vi "UMLEditor_TargetDialog.vi"(6 "SetLastSearchPath(True)":bool=TRUE, 8 "error in (no error)":errorcluster, 10 "Target":string, 11 "GetProjectRefByName":string) -> (0 "error out":errorcluster, 1 "ProjectFolder":path=path "C:/GDS_Test/2009_RT/Test", 2 "ProjectPath":path=path "C:/GDS_Test/2009_RT/Test/Test.lvproj", 3 "TargetIndex":u16, 5 "Targets":string[](array[string]))   [LabVIEW 2016]
uses:
  <resource>/Framework/Providers/Open_GDS/UML/UMLEditor/UMLEditor_StoredPathes.ctl
  <resource>/Framework/Providers/Open_GDS/ClassProviders/Common/File/File_StoredPathesActions.ctl
panel:
  in  "Select":bool
  in  "Target":i32(listbox) caption="Target to use"
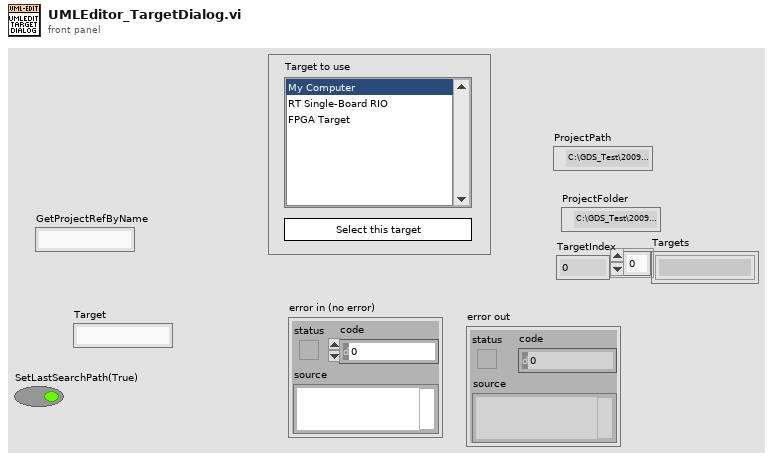
[diagram p1: front panel]
types:
  T1 = typedef "File_StoredPathesActions.ctl" = enum16{"Get Path", "Set Path", "Delete Path", "Clear All Paths"}
  T2 = typedef "UMLEditor_StoredPathes.ctl" = enum16{"LastSearchPath", "QueuedArrayStateVI", "ClassBasePath", "ViTemplatePath", "ApplicationTemplatePath", "IniFilePath", "WizDir", "RevPlugInPath"}
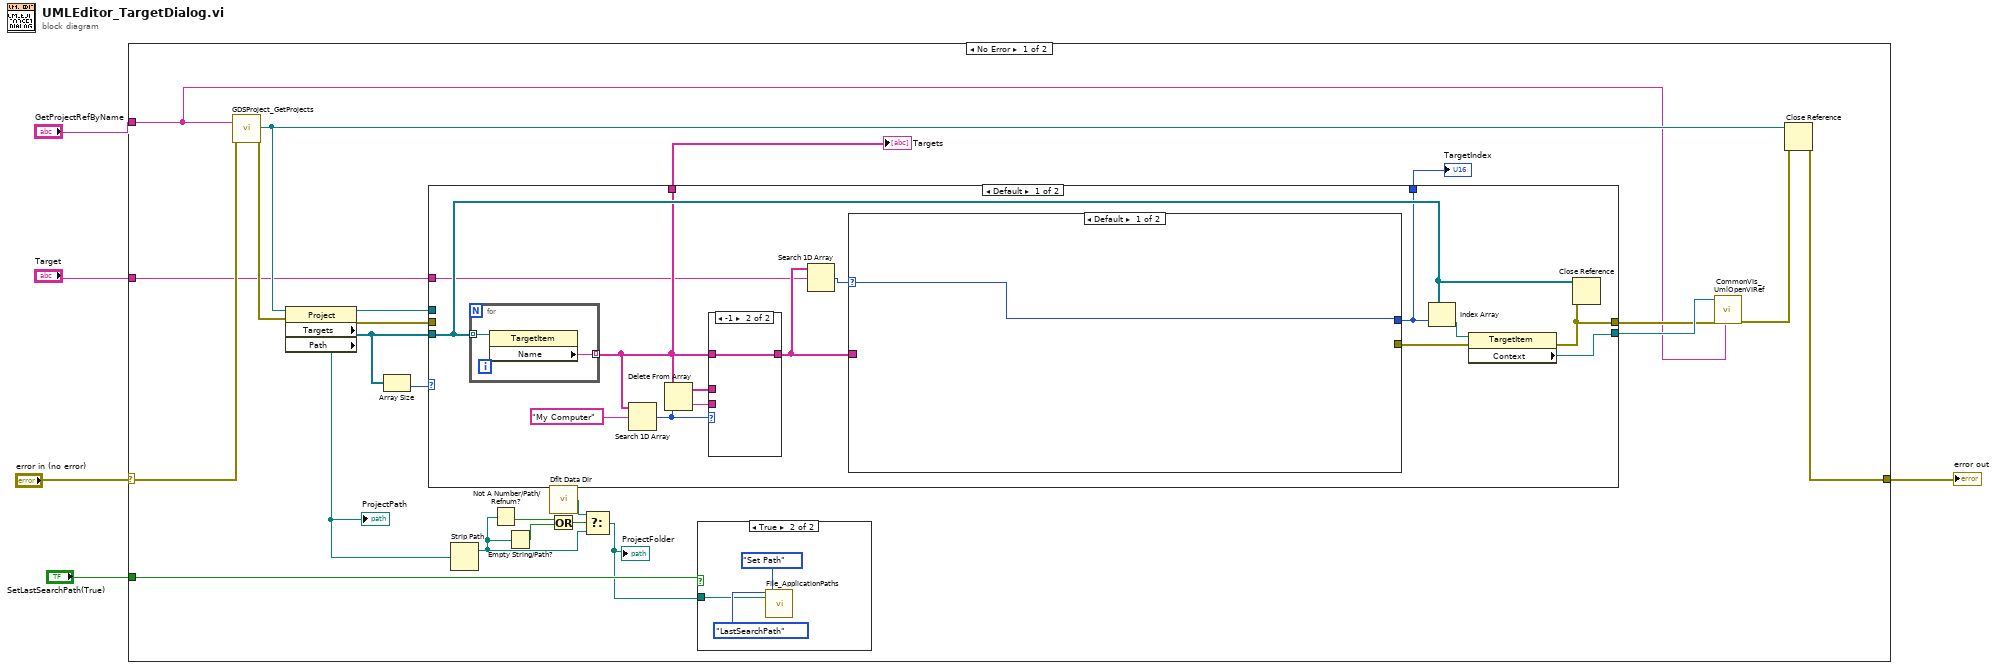
[diagram p0: block diagram]
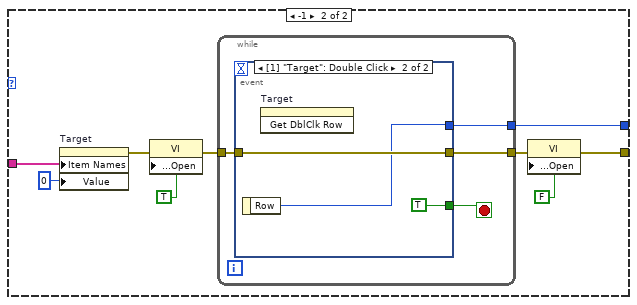
[diagram p3: hidden frame]
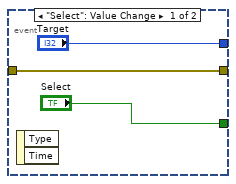
[diagram p4: hidden frame]
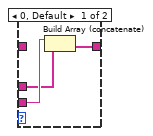
[diagram p5: hidden frame]
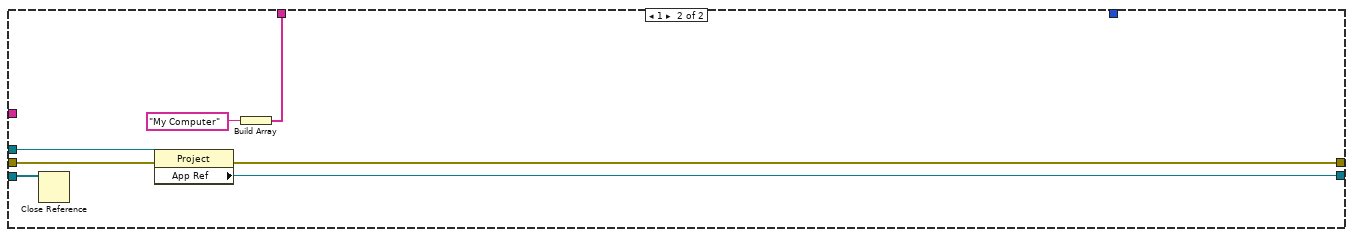
[diagram p6: hidden frame]
diagram:
  n1 = case shown="No Error" "error in (no error)" {
    selector: "error in (no error)" -> [w17 w79]
    tunnel: [w18 w79] -> w5
    tunnel: "GetProjectRefByName" -> [w15 _]
    tunnel: "SetLastSearchPath(True)" -> [w16 _]
    tunnel: "Target" -> [w12 _]
    frame No Error {
      n2 = call <resource>:"GDSProject_GetProjects.vi"("GetProjectRefByName"=w15, "error in (no error)"=w17) -> ("Project Refnum"=w20:refnum<vi>, "error out"=w23:errorcluster)  [unwired: 1 in, 15 out]
      n3 = property class="Project"(reference=w20, error in=w23) -> (reference out=w25:refnum<vi>, error out=w24:errorcluster, "Targets"=w26:refnum<vi>[], "Path"=w19:path)
      "ProjectPath" <- w19
      n4 = Array Size(array=w26) -> (size(s)=w27:i32)
      n5 = case shown="Default" w27 {
        tunnel: w26 -> [w38 w78]
        tunnel: w25 -> [_ w77]
        tunnel: w24 -> [_ w76]
        tunnel: [w40 w75] -> w22
        tunnel: [w39 w74] -> w21
        tunnel: [w36 w72] -> w14
        tunnel: [w35 _] -> w13
        tunnel: w12 -> [w33 _]
        frame Default {
          n6 = for {
            tunnel: w38 -> [w71] mode=indexing
            tunnel: [w70] -> w36 mode=indexing
            n7 = property class="TargetItem"(reference=w71) -> ("Name"=w70:string)  [unwired: 1 in, 2 out]
          }
          n8 = Search 1D Array(1D array=w36, element="My Computer") -> (index of element=w44:i32)  [unwired: 1 in]
          n9 = Delete From Array(array=w36, index=w44) -> (deleted portion=w43:string, array with subset deleted=w37:string[])  [unwired: 1 in]
          n10 = case shown="-1" w44 {
            tunnel: w36 -> [_ w69]
            tunnel: [w67 w69] -> w34
            tunnel: w43 -> [w68 _]
            tunnel: w37 -> [w66 _]
            frame 0, Default {
              n11 = Build Array (concatenate)(w68, w66) -> (w67:string[])
            }
            frame -1 {
            }
          }
          n12 = Search 1D Array(1D array=w34, element=w33) -> (index of element=w32:i32)  [unwired: 1 in]
          n13 = case shown="Default" w32 {
            selector: w32 -> [w46 _]
            tunnel: w34 -> [_ w50]
            tunnel: [_ w48] -> w42
            tunnel: [w46 w47] -> w35
            frame Default {
            }
            frame -1 {
              n14 = property on="Target" class="LstBox (strict)"("Item Names"=w50, "Value"=0 ("Target")) -> (error out=w55:errorcluster)  [unwired: 2 in, 1 out]
              n15 = property class="VI"(error in=w55, "Front Panel.Open"=TRUE ("Front Panel Window:Open")) -> (error out=w53:errorcluster)  [unwired: 1 in, 1 out]
              n16 = while {
                tunnel: w53 -> [w59]
                tunnel: [w58] -> w51
                tunnel: [w57] -> w47
                stop <- w56 stop-if-true
                n17 = event shown="[1] \"Target\": Double Click" {
                  selector: _ -> [_ _]
                  dyn-events: _ -> [_ _]
                  timeout: _ -> [_ _]
                  tunnel: w59 -> [w62 w65]
                  tunnel: [w62 w65] -> w58
                  tunnel: ["Target" w64] -> w57
                  tunnel: ["Select" TRUE ("Select")] -> w56
                  event "Select": Value Change {
                    n18 = event-data() -> ()  [unwired: 1 in, 2 out]
                  }
                  event "Target": Double Click {
                    n19 = event-data() -> ("Row"=w64:i32)  [unwired: 1 in]
                    n20 = invoke on="Target" class="LstBox (strict)" method="Get DblClk Row"() -> ()  [unwired: 3 in, 3 out]
                  }
                }
              }
              n21 = property class="VI"(error in=w51, "Front Panel.Open"=FALSE ("Front Panel Window:Open")) -> (error out=w48:errorcluster)  [unwired: 1 in, 1 out]
            }
          }
          n22 = Index Array(array=w38, index=w35) -> (element=w41:refnum<vi>)
          n23 = property class="TargetItem"(reference=w41, error in=w42) -> (error out=w39:errorcluster, "Context"=w40:refnum<vi>)  [unwired: 1 out]
          n24 = Close Reference(reference=w38, error in (no error)=w39) -> ()  [unwired: 1 out]
        }
        frame 1 {
          n25 = Close Reference(reference=w78) -> ()  [unwired: 1 in, 1 out]
          n26 = property class="Project"(reference=w77, error in=w76) -> (error out=w74:errorcluster, "App Ref"=w75:refnum<vi>)  [unwired: 1 out]
          n27 = Build Array("My Computer" ("element")) -> (w72:string[])
        }
      }
      "Targets" <- w14
      "TargetIndex" <- w13
      n28 = Strip Path(path=w19) -> (stripped path=w7:path)  [unwired: 1 out]
      n29 = Not A Number/Path/Refnum?(number/path/refnum=w7) -> (NaN/Path/Refnum?=w10:bool)
      n30 = Empty String/Path?(string/path=w7) -> (empty?=w11:bool)
      n31 = call <vilib>:"Dflt Data Dir.vi"() -> ("App:Default Data Directory"=w8:path)
      n32 = Or(x=w10, y=w11) -> (x .or. y?=w9:bool)
      n33 = Select(t=w8, s=w9, f=w7) -> (s? t:f=w6:path)
      "ProjectFolder" <- w6
      n34 = case shown="True" w16 {
        tunnel: w6 -> [_ w29]
        frame False {
        }
        frame True {
          n35 = call <resource>:"File_ApplicationPaths.vi"("PathName"=UMLEditor_StoredPathes."LastSearchPath" ("UMLPathes"), "Path In"=w29, "Method (Get Path)"=File_StoredPathesActions."Set Path") -> ()  [unwired: 1 in, 16 out]
        }
      }
      n36 = call <resource>:"CommonVIs_UmlOpenVIRef.vi"("ProjectNameIn"=w15, "error in"=w21, "AppRef"=w22) -> ("error out"=w28:errorcluster)  [unwired: 1 in, 7 out]
      n37 = Close Reference(reference=w20, error in (no error)=w28) -> (error out=w18:errorcluster)
    }
    frame Error {
    }
  }
  "error out" <- w5
